vi "Configure Sweep.vi"(0 "VISA resource name":refnum<visa-resource-name>, 1 "Channel (1)":i32=1, 2 "Number of Measurement Points (201)":i32=201, 3 "Auto Sweep Time (F: Off)":bool, 5 "Sweep Time (0.001)":dbl=0.001 format="%^.3g", 9 "Delay Time (0.001)":dbl=0.001 format="%^.3g", 11 "error in (no error)":errorcluster, 12 "Sweep Mode (0: Stepped)":u16(ring) items=["Stepped", "Fast Stepped Mode"], 13 "Sweep Type (0: Linear Sweep)":u16(ring) items=["Linear Sweep", "Logarithmic Sweep", "Segment Sweep", "Power Sweep", "DC Bias"], 14 "Configure Avoid Mode (F: Off)":bool) -> (4 "VISA resource name out":refnum<visa-resource-name>, 15 "error out":errorcluster)   [LabVIEW 2012, in "Tektronix TTR500 Series.lvlib"]
doc: "This VI configures sweep parameters."
uses:
  <instrlib>/Tektronix TTR500 Series/Tektronix TTR500 Series.lvlib
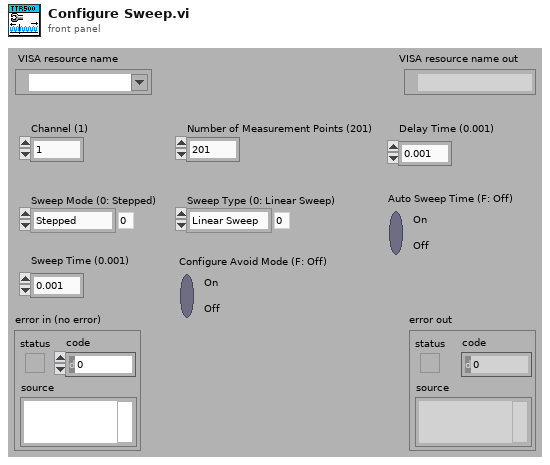
[diagram p1: front panel]
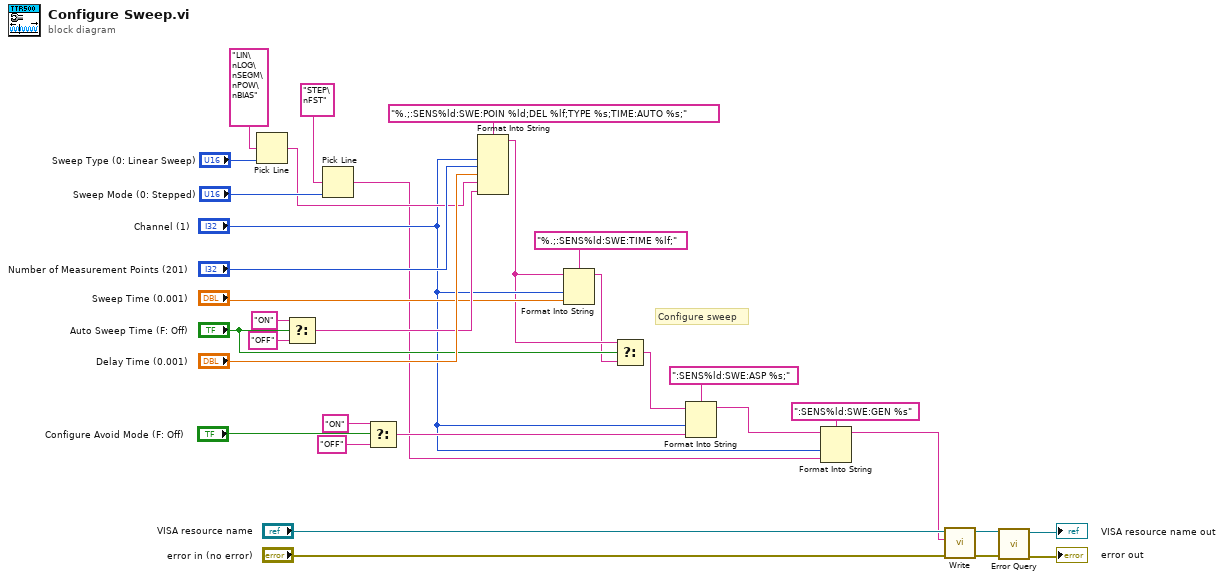
[diagram p0: block diagram]
diagram:
  # "Configure sweep"
  n1 = Pick Line(multi-line string="LIN\nLOG\nSEGM\nPOW\nBIAS", line index="Sweep Type (0: Linear Sweep)") -> (output string=w26:string)  [unwired: 1 in]
  n2 = Select(t="ON", s="Auto Sweep Time (F: Off)", f="OFF") -> (s? t:f=w23:string)
  n3 = Pick Line(multi-line string="STEP\nFST", line index="Sweep Mode (0: Stepped)") -> (output string=w6:string)  [unwired: 1 in]
  n4 = Select(t="ON", s="Configure Avoid Mode (F: Off)", f="OFF") -> (s? t:f=w12:string)
  n5 = Format Into String(format string="%.;:SENS%ld:SWE:POIN %ld;DEL %lf;TYPE %s;TIME:AUTO %s;", "Channel (1)", "Number of Measurement Points (201)", "Delay Time (0.001)", w26, w23) -> (resulting string=w5:string)  [unwired: 2 in, 1 out]
  n6 = Format Into String(format string="%.;:SENS%ld:SWE:TIME %lf;", initial string=w5, "Channel (1)", "Sweep Time (0.001)") -> (resulting string=w4:string)  [unwired: 1 in, 1 out]
  n7 = Select(t=w5, s="Auto Sweep Time (F: Off)", f=w4) -> (s? t:f=w10:string)
  n8 = Format Into String(format string=":SENS%ld:SWE:ASP %s;", initial string=w10, "Channel (1)", w12) -> (resulting string=w9:string)  [unwired: 1 in, 1 out]
  n9 = Format Into String(format string=":SENS%ld:SWE:GEN %s", initial string=w9, "Channel (1)", w6) -> (resulting string=w1:string)  [unwired: 1 in, 1 out]
  n10 = call <instrlib>:"Write.vi"("error in (no error)"="error in (no error)", "String ()"=w1, "VISA resource name"="VISA resource name") -> ("error out"=w18:errorcluster, "VISA resource name out"=w19:refnum<visa-resource-name>)  [unwired: 6 in, 1 out]
  n11 = call <instrlib>:"Error Query.vi"("error in (no error)"=w18, "VISA resource name"=w19) -> ("error out"=→"error out":errorcluster, "VISA resource name out"=→"VISA resource name out":refnum<visa-resource-name>)  [unwired: 6 in, 2 out]
